vi "List Rules as Strings.vi"(8 "error in (no error)":errorcluster, 11 "GlobalLogFilter in":refnum<class "LogFilter.lvclass">) -> (0 "error out":errorcluster, 2 "Rule Strings":string[](array[string]), 3 "GlobalLogFilter out":refnum<class "LogFilter.lvclass">)   [LabVIEW 2017, in "Communicable State Machine.lvlib" / "LogFilter.lvclass"]
doc: "-- <b>Controls</b> --\n- <b>GlobalLogFilter in</b>:\n\n-- <b>Indicators</b> --\n- <b>Rule Strings</b>:\n- <b>GlobalLogFilter out</b>:"
uses:
  LogFilter.lvclass
  LogFilter.lvclass/LogFilter.ctl
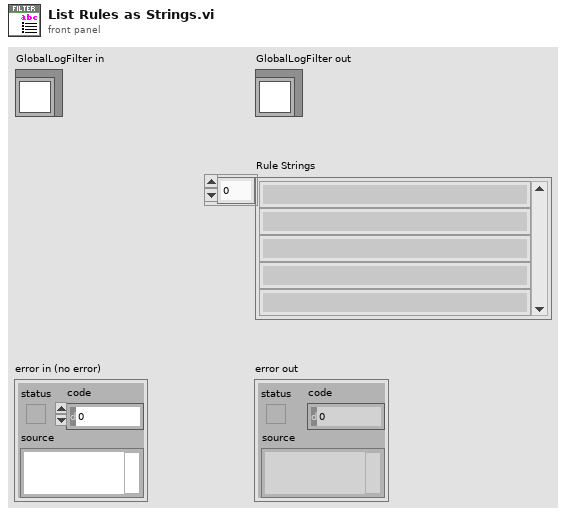
[diagram p1: front panel]
types:
  T1 = typedef "Communicable State Machine.lvlib/_CSM_GlobalLog_MSG_TYPE.ctl" = enum16{"User Log", "State Change", "Status", "Interrupt", "Register", "Unregister", "Error Log", "Module Created", "Module Destroyed"}
  T2 = typedef "Communicable State Machine.lvlib/_CSM_GlobalLog_STATE_TYPE.ctl" = enum16{"State - Internal State", "State - External Message", "State - Response", "State - Complete"}
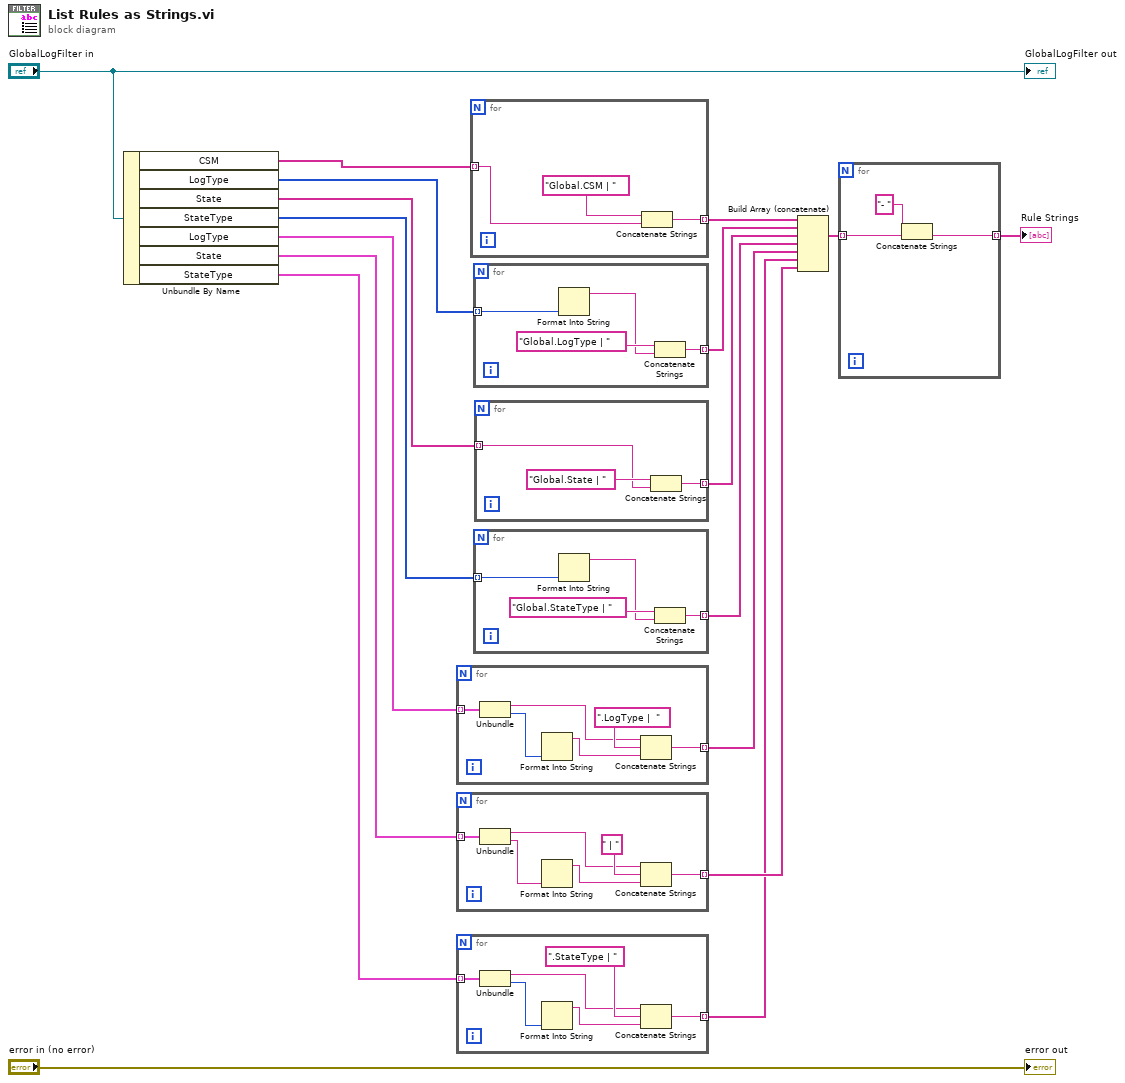
[diagram p0: block diagram]
diagram:
  n1 = Unbundle By Name("GlobalLogFilter in") -> ("CSM"=w16:string[], "LogType"=w14:T1[], "State"=w12:string[], "StateType"=w4:T2[], "LogType"=w10:cluster{"CSM":string, "LogType":T1}[], "State"=w8:cluster{"CSM":string, "State":string}[], "StateType"=w2:cluster{"CSM":string, "LogType":T2}[])
  n2 = for {
    tunnel: w10 -> [w22] mode=indexing
    tunnel: [w23] -> w9 mode=indexing
    n3 = Unbundle(w22) -> ("CSM"=w21:string, "LogType"=w20:T1)
    n4 = Format Into String(w20) -> (resulting string=w19:string)  [unwired: 3 in, 1 out]
    n5 = Concatenate Strings(w21, ".LogType |  " ("string"), w19) -> (w23:string)
  }
  n6 = for {
    tunnel: w8 -> [w28] mode=indexing
    tunnel: [w29] -> w7 mode=indexing
    n7 = Unbundle(w28) -> ("CSM"=w27:string, "State"=w26:string)
    n8 = Format Into String(w26) -> (resulting string=w25:string)  [unwired: 3 in, 1 out]
    n9 = Concatenate Strings(w27, " | " ("string"), w25) -> (w29:string)
  }
  n10 = for {
    tunnel: w2 -> [w34] mode=indexing
    tunnel: [w35] -> w1 mode=indexing
    n11 = Unbundle(w34) -> ("CSM"=w33:string, "LogType"=w32:T2)
    n12 = Format Into String(w32) -> (resulting string=w31:string)  [unwired: 3 in, 1 out]
    n13 = Concatenate Strings(w33, ".StateType | " ("string"), w31) -> (w35:string)
  }
  n14 = for {
    tunnel: w16 -> [w38] mode=indexing
    tunnel: [w37] -> w15 mode=indexing
    n15 = Concatenate Strings("Global.CSM | " ("string"), w38) -> (w37:string)
  }
  n16 = for {
    tunnel: w14 -> [w41] mode=indexing
    tunnel: [w42] -> w13 mode=indexing
    n17 = Format Into String(w41) -> (resulting string=w40:string)  [unwired: 3 in, 1 out]
    n18 = Concatenate Strings("Global.LogType | " ("string"), w40) -> (w42:string)
  }
  n19 = for {
    tunnel: w4 -> [w44] mode=indexing
    tunnel: [w46] -> w3 mode=indexing
    n20 = Format Into String(w44) -> (resulting string=w45:string)  [unwired: 3 in, 1 out]
    n21 = Concatenate Strings("Global.StateType | " ("string"), w45) -> (w46:string)
  }
  n22 = for {
    tunnel: w12 -> [w48] mode=indexing
    tunnel: [w49] -> w11 mode=indexing
    n23 = Concatenate Strings("Global.State | " ("string"), w48) -> (w49:string)
  }
  n24 = Build Array (concatenate)(w15, w13, w11, w3, w9, w1, w7) -> (w5:string[])
  n25 = for {
    tunnel: [w51] -> w6 mode=indexing
    tunnel: w5 -> [w52] mode=indexing
    n26 = Concatenate Strings("- " ("string"), w52) -> (w51:string)
  }
  "Rule Strings" <- w6
  "error out" <- "error in (no error)"
  "GlobalLogFilter out" <- "GlobalLogFilter in"
